vi "test Get Base 16.vi"(11 "Test Case In":refnum<class "test Electronic Datasheet.lvclass">) -> (0 "error out":errorcluster, 3 "Test Case Out":refnum<class "test Electronic Datasheet.lvclass">)   [LabVIEW 2024, in "Test Utilities.lvclass"]
uses:
  Test Utilities.lvclass
  Test Utilities.lvclass/Test Utilities.ctl
  EDS-File-Viewer/Tests/source/test Electronic Datasheet/test Electronic Datasheet.lvclass
  <vilib>/Astemes/LUnit/Test Case.lvclass
  source/CANopen.lvlib
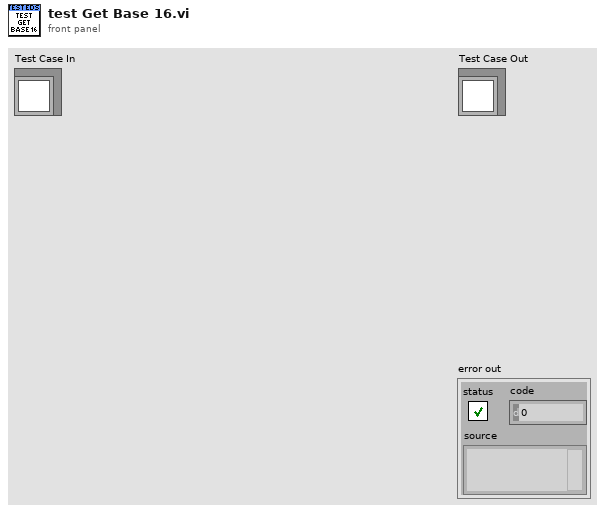
[diagram p1: front panel]
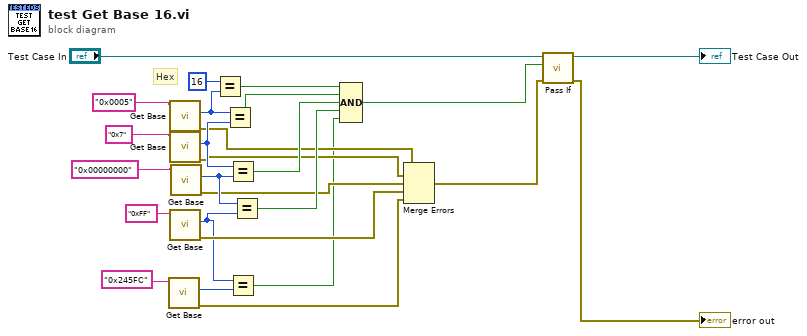
[diagram p0: block diagram]
diagram:
  # "Hex"
  n1 = call "Get Base.vi"("Default Value"="0x245FC") -> ("error out"=w1:errorcluster, "Number Base"=w4:u8)  [unwired: 8 in, 1 out]
  n2 = call "Get Base.vi"("Default Value"="0x0005") -> ("error out"=w7:errorcluster, "Number Base"=w19:u8)  [unwired: 8 in, 1 out]
  n3 = call "Get Base.vi"("Default Value"="0x7") -> ("error out"=w8:errorcluster, "Number Base"=w18:u8)  [unwired: 8 in, 1 out]
  n4 = call "Get Base.vi"("Default Value"="0xFF") -> ("error out"=w10:errorcluster, "Number Base"=w3:u8)  [unwired: 8 in, 1 out]
  n5 = call "Get Base.vi"("Default Value"="0x00000000") -> ("error out"=w9:errorcluster, "Number Base"=w12:u8)  [unwired: 8 in, 1 out]
  n6 = Equal?(x=u8 16, y=w19) -> (x = y?=w17:bool)
  n7 = Equal?(x=w19, y=w18) -> (x = y?=w16:bool)
  n8 = Equal?(x=w18, y=w12) -> (x = y?=w15:bool)
  n9 = Equal?(x=w3, y=w4) -> (x = y?=w2:bool)
  n10 = Equal?(x=w12, y=w3) -> (x = y?=w11:bool)
  n11 = Compound Arithmetic op=AND(w17, w16, w15, w11, w2) -> (w14:bool)
  n12 = Merge Errors(w7, w8, w9, w10, w1) -> (w6:errorcluster)
  n13 = call <vilib>:"Pass If.vi"("error in (no error)"=w6, "Pass?"=w14, "LUnit Test Case In"="Test Case In") -> ("error out"=→"error out":errorcluster, "LUnit Test Case Out"=→"Test Case Out":refnum<class "test Electronic Datasheet.lvclass">)  [unwired: 7 in]
